vi "LabelLanguageUpdate.vi"(10 "Language":T1, 11 "Array":refnum<vi>[](array[refnum])) -> ()   [LabVIEW 2020]
uses:
  Controls/Language Enum.ctl
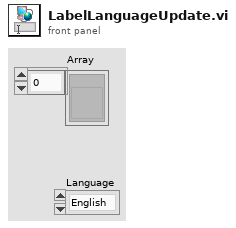
[diagram p1: front panel]
types:
  T1 = typedef "Language Enum.ctl" = enum16{"English", "Español", "Français"}
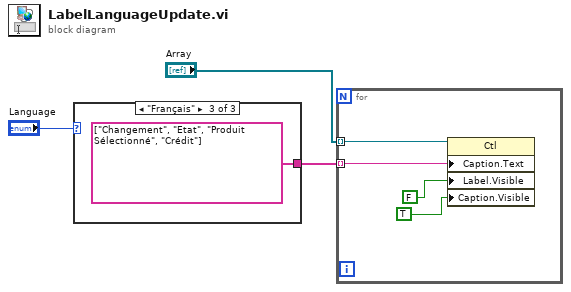
[diagram p0: block diagram]
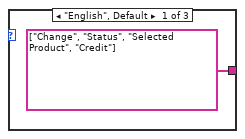
[diagram p2: hidden frame]
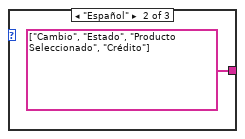
[diagram p3: hidden frame]
diagram:
  n1 = case shown="\"Français\"" "Language" {
    tunnel: [string[] ["Change", "Status", "Selected Product", "Credit"] string[] ["Cambio", "Estado", "Producto Seleccionado", "Crédito"] string[] ["Changement", "Etat", "Produit Sélectionné", "Crédit"]] -> w1
    frame "English", Default {
    }
    frame "Español" {
    }
    frame "Français" {
    }
  }
  n2 = for {
    tunnel: "Array" -> [w10] mode=indexing
    tunnel: w1 -> [w9] mode=indexing
    n3 = property class="Ctl"(reference=w10, "Caption.Text"=w9, "Label.Visible"=FALSE, "Caption.Visible"=TRUE) -> ()  [unwired: 1 in, 2 out]
  }
